vi "startUp.vi"(8 "error in (no error)":errorcluster, 9 "Pane":refnum<vi>, 10 "Path":path, 11 "ICSettingsViewer in":refnum<class "ICSettingsViewer.lvclass">) -> (0 "error out":errorcluster, 1 "Pane out":refnum<vi>, 3 "ICSettingsViewer out":refnum<class "ICSettingsViewer.lvclass">)   [LabVIEW 2009, in "Views.lvlib" / "Camera.lvlib" / "ICSettingsViewer.lvclass"]
uses:
  ICSettingsViewer.lvclass
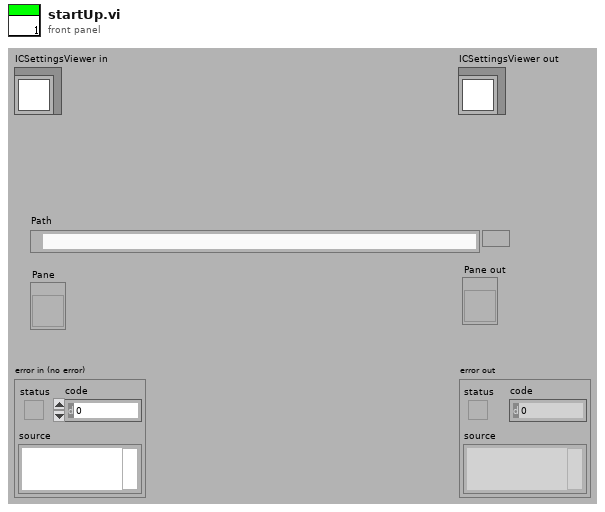
[diagram p1: front panel]
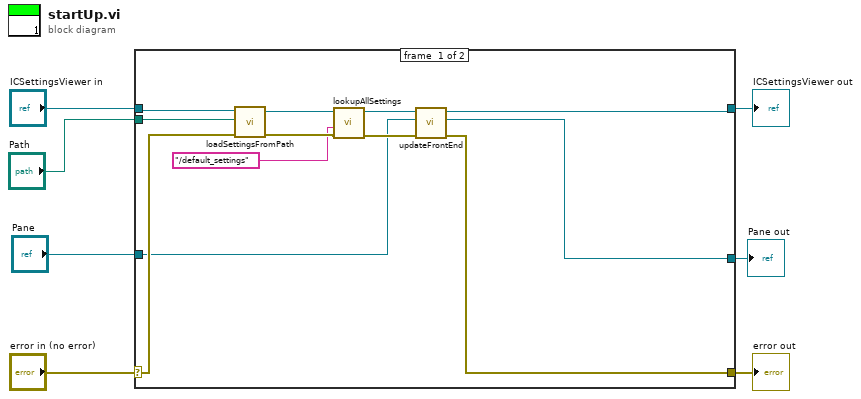
[diagram p0: block diagram]
diagram:
  n1 = case shown="No Error" "error in (no error)" {
    selector: "error in (no error)" -> [w18 w21]
    tunnel: [w10 w21] -> w6
    tunnel: [w12 w20] -> w4
    tunnel: "ICSettingsViewer in" -> [w19 w20]
    tunnel: "Path" -> [w17 _]
    tunnel: "Pane" -> [w9 _]
    tunnel: [w8 _] -> w1
    frame #0 {
      n2 = call "loadSettingsFromPath.vi"("error in (no error)"=w18, "Path"=w17, "ICSettingsViewer in"=w19) -> ("error out"=w15:errorcluster, "ICSettingsViewer out"=w16:refnum<class "ICSettingsViewer.lvclass">)  [unwired: 7 in]
      n3 = call "lookupAllSettings.vi"("error in (no error)"=w15, "whichSettings"="/default_settings", "ICSettingsViewer in"=w16) -> ("error out"=w11:errorcluster, "ICSettingsViewer out"=w13:refnum<class "ICSettingsViewer.lvclass">)  [unwired: 7 in]
      n4 = call "updateFrontEnd.vi"("error in (no error)"=w11, "Pane"=w9, "ICSettingsViewer in"=w13) -> ("error out"=w10:errorcluster, "Pane out"=w8:refnum<vi>, "ICSettingsViewer out"=w12:refnum<class "ICSettingsViewer.lvclass">)  [unwired: 6 in]
    }
    frame #1 {
    }
  }
  "error out" <- w6
  "ICSettingsViewer out" <- w4
  "Pane out" <- w1
